vi "crop.vi"(8 "boxsize":i32, 9 "Y":dbl, 10 "X":dbl, 11 "Data 16":u16[][](array[numeric])) -> (3 "Array":u16[][](array[numeric]))   [LabVIEW 2015]
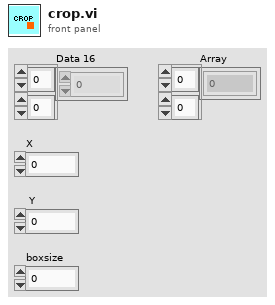
[diagram p1: front panel]
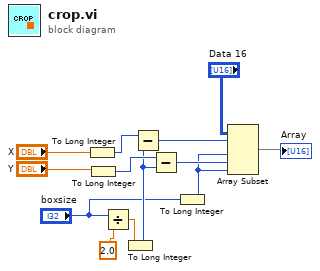
[diagram p0: block diagram]
diagram:
  n1 = To Long Integer(number="X") -> (32bit integer=w12:i32)
  n2 = To Long Integer(number="Y") -> (32bit integer=w13:i32)
  n3 = Divide(x="boxsize", y=2.0) -> (x/y=w5:dbl)
  n4 = To Long Integer(number=w5) -> (32bit integer=w4:i32)
  n5 = Subtract(x=w12, y=w4) -> (x-y=w7:i32)
  n6 = Subtract(x=w13, y=w4) -> (x-y=w3:i32)
  n7 = To Long Integer(number="boxsize") -> (32bit integer=w1:i32)
  n8 = Array Subset(array="Data 16", index (row)=w7, length (row)=w1, index (col)=w3, length (col)=w1) -> (→"Array":u16[][])
